vi "TPG261_ReadData.vi"(7 "Baud Rate":u32(ring) items=["9600 (default)", "19200", "38400", "57600", "115200"], 8 "error in (no error)":errorcluster caption="Fehler (Eingang, kein Fehler)", 11 "input refnum":refnum<visa-resource-name> caption="ComPort") -> (0 "error out":errorcluster)   [LabVIEW 2012]
doc: "This VI is an example of how to use the PV ActiveLine subVIs programmatically. This VI first initializes the instrument, takes measurements, then closes the instrument."
uses:
  <instrlib>/PV ActiveLine/Public/Configure/PV ActiveLine - FullScaleRange (TPG361).vi
  <instrlib>/PV ActiveLine/Public/Configure/PV ActiveLine - FilterTime (TPG361).vi
  <instrlib>/PV ActiveLine/Public/Configure/PV ActiveLine - CalibrationFactor (TPG361).vi
  <instrlib>/PV ActiveLine/PV ActiveLine.lvlib
panel:
  out "SP1-Params":string
  out "gaugeStatus":string
  out "gaugeID":string
  out "Gauge out":string[](array[string])
  out "Get Calibration factor 1":dbl=0.000753 format="%.3f"
  out "Sensor 1 Get":i8(ring)=3 items=["0.01 mbar", "0.1 mbar", "1 mbar", "10 mbar", "100 mbar", "1000 mbar", "2 bar", "5 bar", "10 bar", "50 bar"]
  out "Sensor 1 Get 2":i8(ring)=2 items=["Filter off", "fast", "normal", "slow"]
  out "Unit Get":i8(ring) items=["mbar / bar", "Torr", "Pascal", "Micron", "hPascal (default)", "Volt"]
  in  "Unit Set":i8(ring) items=["mbar / bar", "Torr", "Pascal", "Micron", "hPascal (default)", "Volt"]
  in  "W/R":bool
  out "Status Sensor 1":i32(ring) items=["data OK", "underrange", "overrange", "sensor error", "sensor off", "no sensor", "ID error"]
  out "Pressure Sensor 1":dbl format="%.3e"
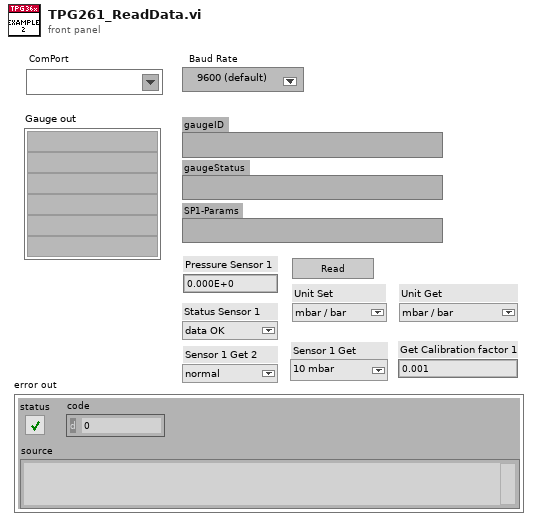
[diagram p1: front panel]
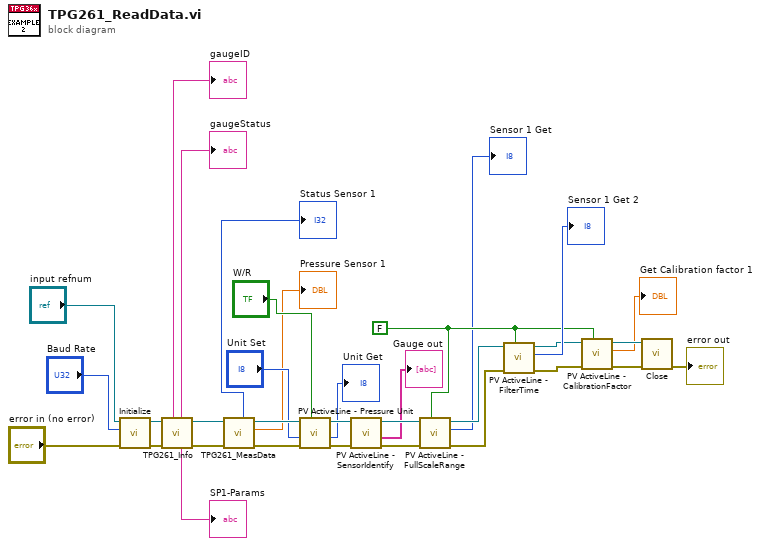
[diagram p0: block diagram]
diagram:
  w13 = FALSE ("W/R")
  n1 = call <instrlib>:"Initialize.vi"("error in (no error)"="error in (no error)", "Baud Rate"="Baud Rate", "input refnum"="input refnum") -> ("Cluster (Ausgang)"=w7:errorcluster, "Referenz out"=w6:refnum<visa-resource-name>)  [unwired: 7 in]
  n2 = call "TPG261_Info.vi"("error in (no error)"=w7, "input refnum"=w6) -> ("error out"=w1:errorcluster, "ComPort out"=w5:refnum<visa-resource-name>, "SP1-Params"=→"SP1-Params":string, "gaugeStatus"=→"gaugeStatus":string, "gaugeID"=→"gaugeID":string)  [unwired: 5 in]
  n3 = call "TPG261_MeasData.vi"("Fehler (Eingang)"=w1, "Referenz in"=w5) -> ("Cluster (Ausgang)"=w29:errorcluster, "Pressure CH1"=→"Pressure Sensor 1":dbl, "Referenz out"=w30:refnum<visa-resource-name>, "Status CH1"=→"Status Sensor 1":i32)  [unwired: 6 in]
  n4 = call <instrlib>:"PV ActiveLine - Pressure Unit.vi"("W/R"="W/R", "Fehler (Eingang)"=w29, "Unit Set"="Unit Set", "Referenz in"=w30) -> ("Cluster (Ausgang)"=w26:errorcluster, "Unit Get"=→"Unit Get":i8, "Referenz out"=w27:refnum<visa-resource-name>)  [unwired: 5 in]
  n5 = call <instrlib>:"PV ActiveLine - SensorIdentify.vi"("Fehler (Eingang)"=w26, "Referenz in"=w27) -> ("Cluster (Ausgang)"=w15:errorcluster, "Gauge out"=→"Gauge out":string[], "Referenz out"=w17:refnum<visa-resource-name>)  [unwired: 7 in]
  n6 = call-poly <instrlib>:"PV ActiveLine - FullScaleRange.vi"("W/R"=w13, "Fehler (Eingang)"=w15, "Referenz in"=w17) -> ("Cluster (Ausgang)"=w14:errorcluster, "Sensor 1 Get"=→"Sensor 1 Get":i8, "Referenz out"=w16:refnum<visa-resource-name>)  [unwired: 6 in]
  n7 = call-poly <instrlib>:"PV ActiveLine - FilterTime.vi"("W/R"=w13, "Fehler (Eingang)"=w14, "Referenz in"=w16) -> ("Cluster (Ausgang)"=w19:errorcluster, "Sensor 1 Get"=→"Sensor 1 Get 2":i8, "Referenz out"=w21:refnum<visa-resource-name>)  [unwired: 6 in]
  n8 = call-poly <instrlib>:"PV ActiveLine - CalibrationFactor.vi"("W/R"=w13, "Fehler (Eingang)"=w19, "Referenz in"=w21) -> ("Cluster (Ausgang)"=w18:errorcluster, "Get Calibration factor"=→"Get Calibration factor 1":dbl, "Referenz out"=w20:refnum<visa-resource-name>)  [unwired: 6 in]
  n9 = call <instrlib>:"Close.vi"("error in (no error)"=w18, "VISA resource name"=w20) -> ("error out"=→"error out":errorcluster)  [unwired: 9 in]
